vi "Target FF Trajectory Manager.vi"(7 "Error":dbl, 8 "Phase":dbl, 9 "Learning Gains":T1={"KL"=15.0, "Beta"=0.97, "D"=18}, 11 "HS":bool) -> (0 "Error Out":errorcluster)   [LabVIEW 2018, in "COBRA Iterative Learning Control Library.lvlib"]
uses:
  COBRA Iterative Learning Control Library.lvlib
  Target Learning Gains.ctl
panel:
  out "UFF Table":dbl[](array[numeric])
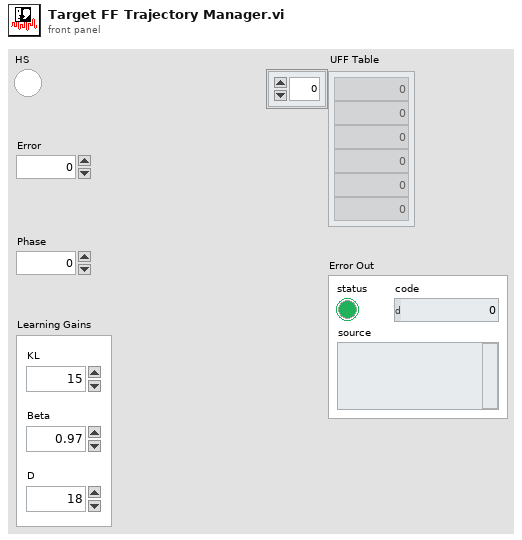
[diagram p1: front panel]
types:
  T1 = typedef "COBRA Iterative Learning Control Library.lvlib/Target Learning Gains.ctl" = cluster{"KL":dbl, "Beta":dbl, "D":i32}
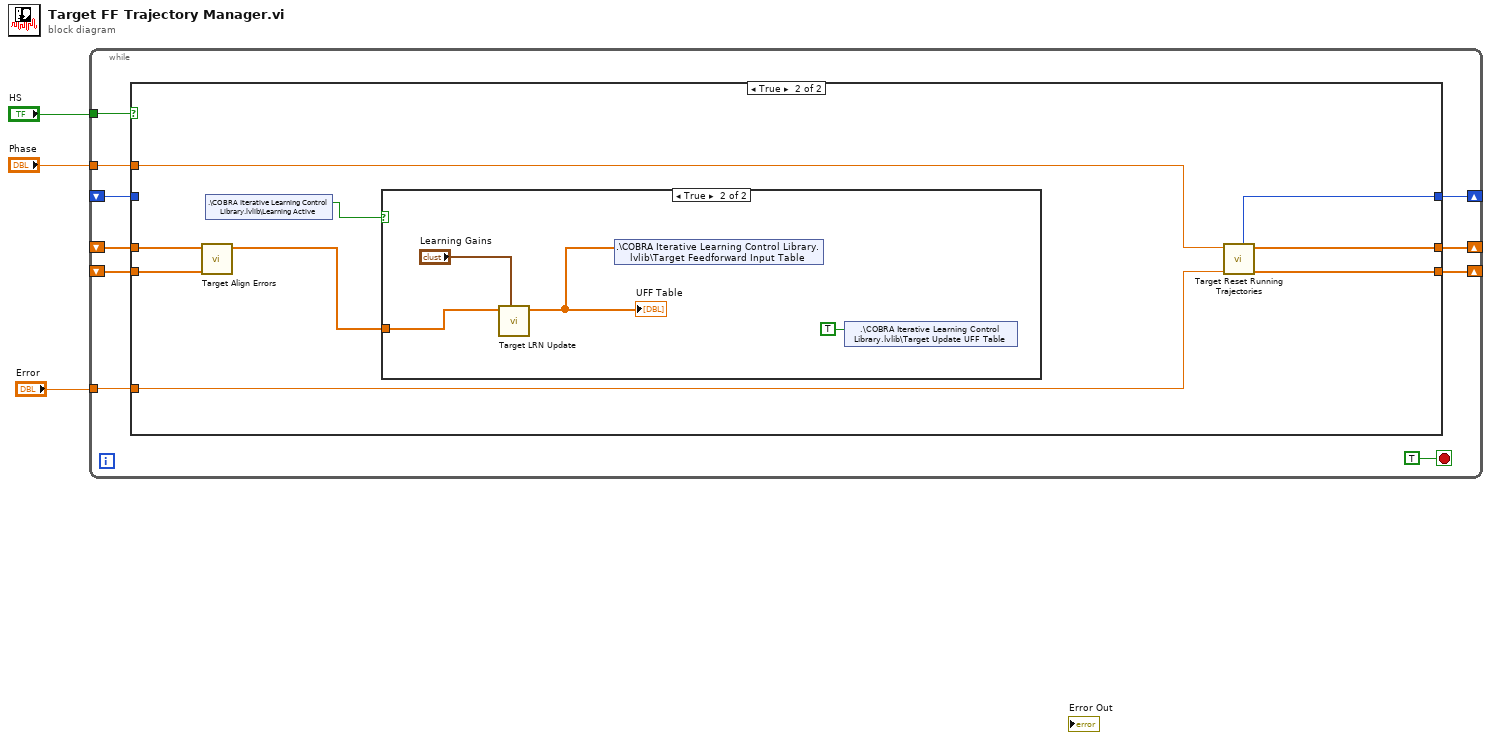
[diagram p0: block diagram]
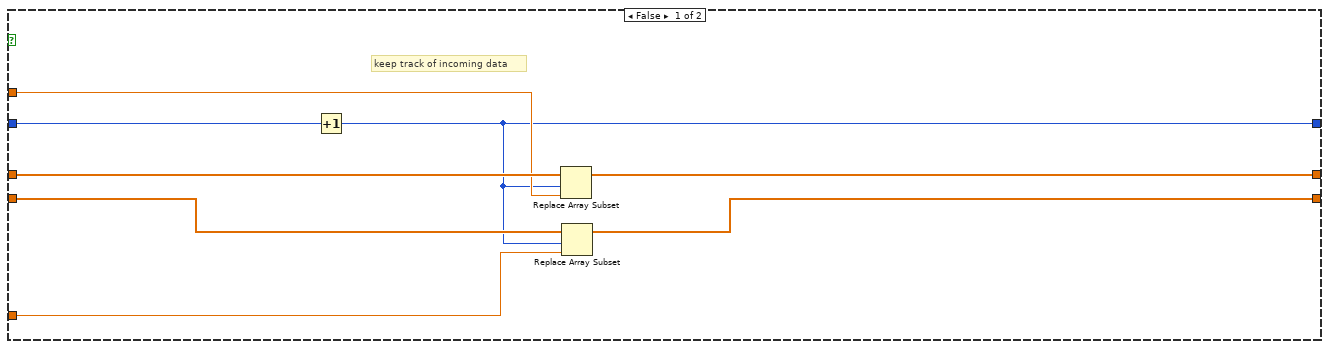
[diagram p2: hidden frame]
diagram:
  n1 = while {
    tunnel: "HS" -> [w12]
    tunnel: "Phase" -> [w11]
    tunnel: "Error" -> [w10]
    shift-right: [w9] -> _
    shift-left: _ -> [w4]
    shift-right: [w8] -> _
    shift-left: _ -> [w6]
    shift-right: [w7] -> _
    shift-left: _ -> [w5]
    stop <- TRUE stop-if-true
    n2 = case shown="True" w12 {
      tunnel: w11 -> [w18 w27]
      tunnel: w10 -> [w19 w26]
      tunnel: [w16 w24] -> w9
      tunnel: [w17 w25] -> w8
      tunnel: [w15 w23] -> w7
      tunnel: w6 -> [w21 w30]
      tunnel: w5 -> [w14 _]
      tunnel: w4 -> [w20 w29]
      frame False {
        # "keep track of incoming data"
        n3 = Increment(x=w14) -> (x+1=w15:i32)
        n4 = Replace Array Subset "Replace Array Subset"(array=w21, new element=w18, index=w15) -> (w17:dbl[])
        n5 = Replace Array Subset "Replace Array Subset"(array=w20, new element=w19, index=w15) -> (w16:dbl[])
      }
      frame True {
        n6 = call "Target Align Errors.vi"("Running Error Array"=w29, "Running Phase Array"=w30) -> ("Error Table"=w28:dbl[])  [unwired: 8 in, 1 out]
        n7 = shared-variable ".\\COBRA Iterative Learning Control Library.lvlib\\Learning Active"() -> (w22:bool)  [unwired: 1 in, 1 out]
        n8 = case shown="True" w22 {
          tunnel: w28 -> [_ w32]
          frame False {
          }
          frame True {
            n9 = call "Target LRN Update.vi"("Learning Gains"="Learning Gains", "Error Lookup Table"=w32) -> ("Updated Feedforward Lookup Table"=w34:dbl[])  [unwired: 9 in]
            "UFF Table" <- w34
            n10 = shared-variable ".\\COBRA Iterative Learning Control Library.lvlib\\Target Feedforward Input Table"(w34) -> ()  [unwired: 1 in, 1 out]
            n11 = shared-variable ".\\COBRA Iterative Learning Control Library.lvlib\\Target Update UFF Table"(TRUE ("Update Lookup Tables")) -> ()  [unwired: 1 in, 1 out]
          }
        }
        n12 = call "Target Reset Running Trajectories.vi"("Error"=w26, "Phase"=w27) -> ("Running Error"=w24:dbl[], "Running Phase"=w25:dbl[], "index"=w23:i32)  [unwired: 7 in]
      }
    }
  }
